vi "main.vi"() -> ()   [LabVIEW 2020]
doc: "This VI demonstrates how to use dynamic events between two VIs. The \"main.vi\" sends a reference for it's \"Fire Event?\" boolean control and a reference for its \"Stop\" button boolean control to the SubVI named \"sub.vi.\" The \"sub.vi\" uses those references to register two dynamic events. Those two dynamic events each have a corresponding event case in the event structure. \n\nIf the \"Fire Event?\" control is set to true in \"main.vi\", the \"Event Fired?\" indicator in \"sub.vi\" lights up. Also if the \"Stop control is set to true in \"main.vi\", both the \"main.vi\" and the \"sub.vi\" are stopped.\n\nUse this example to get you started with using one VI to generate events in a second VI."
panel:
  in  "Cluster":T1
  in  "Numeric":dbl
  in  "stop":bool
  in  "Fire Event?":bool
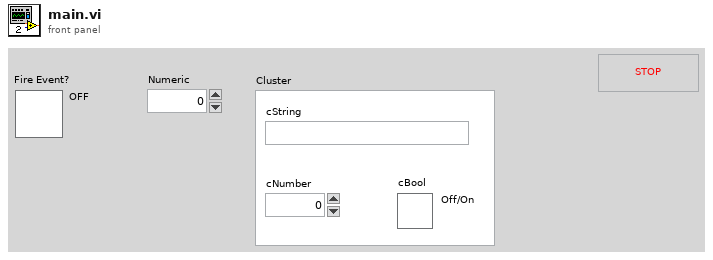
[diagram p1: front panel]
types:
  T1 = cluster{"cString":string, "cNumber":dbl, "cBool":bool}
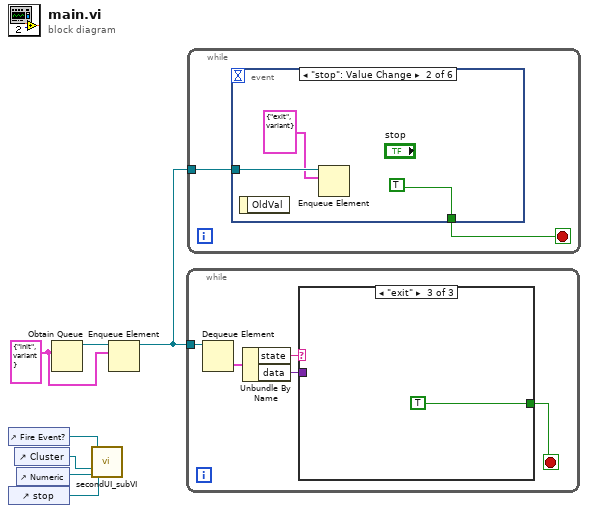
[diagram p0: block diagram]
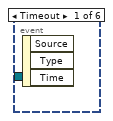
[diagram p2: hidden frame]
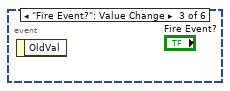
[diagram p3: hidden frame]
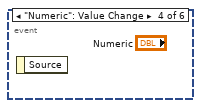
[diagram p4: hidden frame]
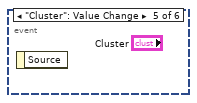
[diagram p5: hidden frame]
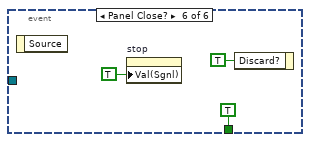
[diagram p6: hidden frame]
diagram:
  w4 = cluster{"state":string, "data":variant} {"state"="init", "data"=variant}
  n1 = control-ref of="Fire Event?"() -> (w6:refnum<vi>)
  n2 = control-ref of="stop"() -> (w7:refnum<vi>)
  n3 = control-ref of="Cluster"() -> (w1:refnum<vi>)
  n4 = control-ref of="Numeric"() -> (w2:refnum<vi>)
  n5 = Obtain Queue(element data type=w4) -> (queue out=w5:refnum<queue>)  [unwired: 4 in, 2 out]
  n6 = call "secondUI_subVI.vi"("Bool Refnum"=w6, "Cluster1"=w1, "Numeric"=w2, "Stop Refnum"=w7) -> ()  [unwired: 12 in]
  n7 = Enqueue Element(queue=w5, element=w4) -> (queue out=w3:refnum<queue>)  [unwired: 2 in, 2 out]
  n8 = while {
    tunnel: w3 -> [w12]
    stop <- w8 stop-if-true
    n9 = Dequeue Element(queue=w12) -> (element=w11:cluster{"state":string, "data":variant})  [unwired: 2 in, 3 out]
    n10 = Unbundle By Name(w11) -> ("state"=w10:string, "data"=w9:variant)
    n11 = case shown="\"exit\"" w10 {
      tunnel: w9 -> [_ _ _]
      tunnel: [_ _ TRUE] -> w8
      frame "", Default {
      }
      frame "init" {
      }
      frame "exit" {
      }
    }
  }
  n12 = while {
    tunnel: w3 -> [w14]
    stop <- w15 stop-if-true
    n13 = event shown="[1] \"stop\": Value Change" {
      selector: _ -> [_ _ _ _ _ _]
      dyn-events: _ -> [_ _ _ _ _ _]
      timeout: _ -> [_ _ _ _ _ _]
      tunnel: [_ TRUE ("stop") _ _ _ TRUE ("stop")] -> w15
      tunnel: w14 -> [_ w17 _ _ _ _]
      event Timeout {
        n14 = event-data() -> ()  [unwired: 1 in, 3 out]
      }
      event "stop": Value Change {
        n15 = event-data() -> ()  [unwired: 1 in, 1 out]
        n16 = Enqueue Element(queue=w17, element=cluster{"state":string, "data":variant} {"state"="exit", "data"=variant}) -> ()  [unwired: 2 in, 3 out]
      }
      event "Fire Event?": Value Change {
        n17 = event-data() -> ()  [unwired: 1 in, 1 out]
      }
      event "Numeric": Value Change {
        n18 = event-data() -> ()  [unwired: 1 in, 1 out]
      }
      event "Cluster": Value Change {
        n19 = event-data() -> ()  [unwired: 1 in, 1 out]
      }
      event Panel Close? {
        n20 = event-data() -> ()  [unwired: 1 in, 1 out]
        n21 = property on="stop" class="Bool"("Val(Sgnl)"=TRUE) -> ()  [unwired: 2 in, 2 out]
        n22 = event-data("Discard?"=TRUE) -> ()  [unwired: 1 in, 1 out]
      }
    }
  }
